vi "Insert Module Channels.vi"(7 "Number of channels":i32, 9 "First channel":i32, 10 "Module":i32, 11 "Channels map":T1(c390)) -> (3 "Channels map out":T1(c390))   [LabVIEW 2024]
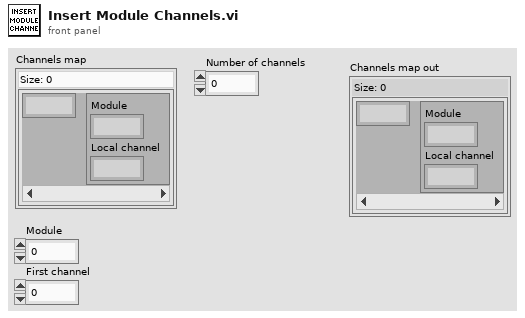
[diagram p1: front panel]
types:
  T1 = map{i32, cluster{"Module":i32, "Local channel":i32}}
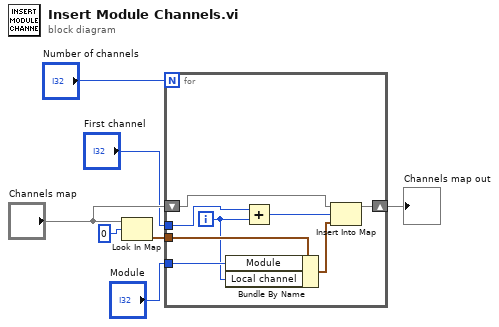
[diagram p0: block diagram]
diagram:
  n1 = Look In Map(map="Channels map", key=0) -> (value=w6:cluster{"Module":i32, "Local channel":i32})  [unwired: 1 in, 1 out]
  n2 = for {
    N: "Number of channels" -> [_]
    tunnel: w6 -> [w14]
    tunnel: "Module" -> [w13]
    shift-right: [w11] -> w4
    shift-left: "Channels map" -> [w15]
    tunnel: "First channel" -> [w10]
    i -> [w9]
    n3 = Bundle By Name(cluster=w14, "Module"=w13, "Local channel"=w9) -> (w12:cluster{"Module":i32, "Local channel":i32})
    n4 = Add(x=w10, y=w9) -> (x+y=w8:i32)
    n5 = Insert Into Map(map in=w15, key=w8, value=w12) -> (map out=w11:T1)  [unwired: 2 out]
  }
  "Channels map out" <- w4
